vi "Q8381 LEVEL SCALE_LEVEL SCALE.vi"(1 "scale":u16(ring) items=["10dB/D", "5dB/D", "2dB/D", "1dB/D", "0.5dB/D", "0.2dB/D"], 2 "GPIB Address":u16=8 max=31 step=1, 3 "VISA resource name":refnum<visa-resource-name>) -> (0 "GPIB Status":bool)   [LabVIEW 2017]
doc: "scale: 0: 10dB/D, 1: 5dB/D,\n 2: 2dB/D, 3: 1dB/D,\n 4: 0.5dB/D, 5: 0.2dB/D."
panel:
  out "Program Code":string
  # "SET LEVEL SCALE"
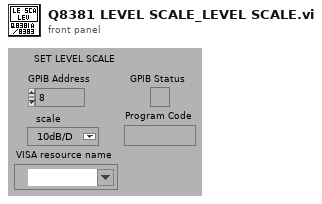
[diagram p1: front panel]
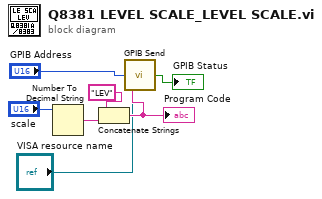
[diagram p0: block diagram]
diagram:
  n1 = Number To Decimal String(number="scale") -> (decimal integer string=w6:string)  [unwired: 1 in]
  n2 = Concatenate Strings("LEV", w6) -> (w4:string)
  "Program Code" <- w4
  n3 = call "GPIB Send.vi"("Command String"=w4, "Address"="GPIB Address", "VISA resource name"="VISA resource name") -> ("Error"=→"GPIB Status":bool)
